vi "Create Channel Buffer.vi"(8 "error in":errorcluster, 10 "Channel":string, 11 "Buffer Lossless DBL in":refnum<class "Buffer Lossless DBL.lvclass">) -> (0 "error out":errorcluster, 3 "Buffer Lossless DBL out":refnum<class "Buffer Lossless DBL.lvclass">)   [LabVIEW 2024, in "Buffer Lossless DBL.lvclass"]
uses:
  Buffer Lossless DBL.lvclass
  Buffer Lossless DBL.lvclass/Buffer Lossless DBL.ctl
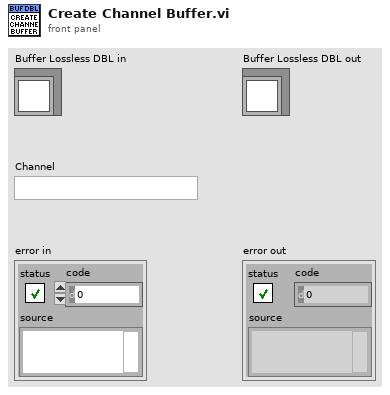
[diagram p1: front panel]
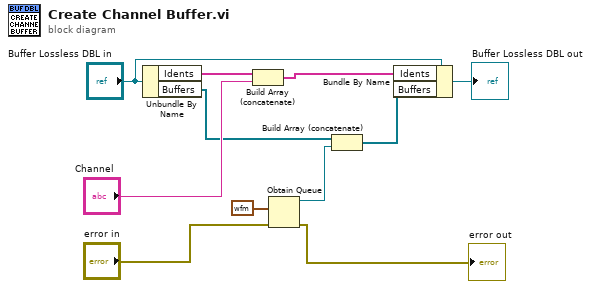
[diagram p0: block diagram]
diagram:
  n1 = Unbundle By Name("Buffer Lossless DBL in") -> ("Idents"=w5:string[], "Buffers"=w6:refnum<queue>[])
  n2 = Build Array (concatenate)(w5, "Channel") -> (w4:string[])
  n3 = Obtain Queue(element data type=waveform(dbl) {"t0"=timestamp(0 s since 1904-01-01), "dt"=1.0, "Y"=[]} ("Waveform"), error in (no error)="error in") -> (queue out=w2:refnum<queue>, error out=→"error out":errorcluster)  [unwired: 3 in, 1 out]
  n4 = Build Array (concatenate)(w6, w2) -> (w3:refnum<queue>[])
  n5 = Bundle By Name(cluster="Buffer Lossless DBL in", "Idents"=w4, "Buffers"=w3) -> (→"Buffer Lossless DBL out":refnum<class "Buffer Lossless DBL.lvclass">)
